vi "KM_file - read-write - list of lines.vi"(7 "read/write control":T1, 9 "header":string, 10 "list of lines IN":string[](array[string]), 11 "file path":path=path "\\\\rus-one\\newdata/data/Ultrasound/Experiment/ProbeTest/Probe10/Hg1201-6-C185-550Cair-3c-83K/sweep3/9w/3366_a.dat") -> (1 "header OUT":string, 2 "list of lines OUT":string[](array[string]))   [LabVIEW 2015]
uses:
  file -- read-write control.ctl
  <vilib>/Utility/file.llb/Read From Spreadsheet File (string).vi
  <vilib>/Utility/file.llb/Write To Spreadsheet File (string).vi
  <vilib>/Utility/file.llb/Write Delimited Spreadsheet (string).vi
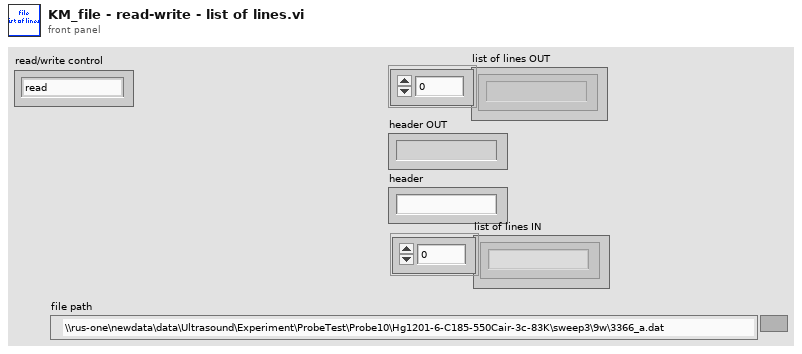
[diagram p1: front panel]
types:
  T1 = typedef "file -- read-write control.ctl" = enum16{"read", "write all", "append one line"}
  T2 = enum16{"open", "replace", "create", "open or create", "replace or create", "replace or create with confirmation"}
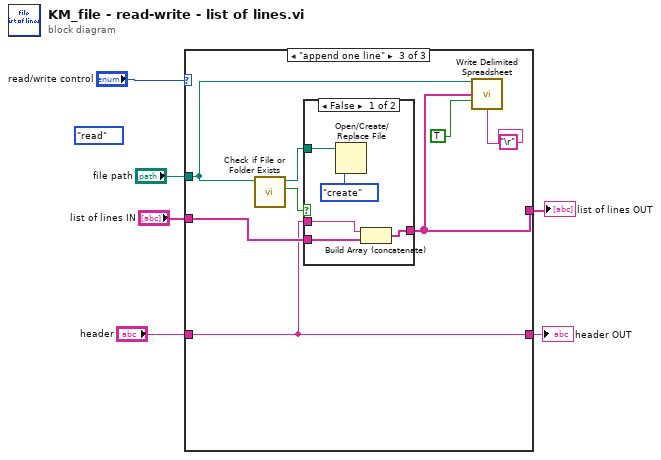
[diagram p0: block diagram]
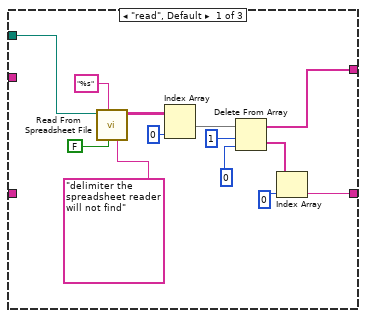
[diagram p2: hidden frame]
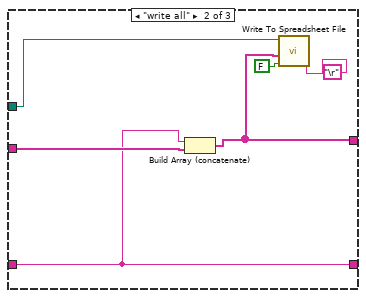
[diagram p3: hidden frame]
diagram:
  (unwired) file_--_read-write_control."read" ("read/write control")
  n1 = case shown="\"append one line\"" "read/write control" {
    tunnel: "file path" -> [w12 w23 w30]
    tunnel: [w8 w21 w26] -> w5
    tunnel: [w7 w20 w28] -> w4
    tunnel: "header" -> [_ w20 w28]
    tunnel: "list of lines IN" -> [_ w22 w29]
    frame "read", Default {
      n2 = call-poly <vilib>:"Read From Spreadsheet File.vi"("delimiter (\\t)"="delimiter the spreadsheet reader will not find" ("delimiter (\\t)"), "transpose (no:F)"=FALSE ("append to file? (new file:F)"), "format (%s)"="%s", "file path (dialog if empty)"=w12) -> ("all rows"=w17:string[][])  [unwired: 3 in, 4 out]
      n3 = Index Array(array=w17, index (col)=0 ("disabled index (col)")) -> (element=w15:string[])  [unwired: 1 in]
      n4 = Delete From Array(array=w15, length=1, index=0) -> (deleted portion=w10:string[], array with subset deleted=w8:string[])
      n5 = Index Array(array=w10, index=0 ("disabled index (col)")) -> (element=w7:string)
    }
    frame "write all" {
      n6 = Build Array (concatenate)(w20, w22) -> (w21:string[])
      n7 = call-poly <vilib>:"Write To Spreadsheet File.vi"("delimiter (\\t)"="\r", "append to file? (new file:F)"=FALSE, "1D data"=w21, "file path (dialog if empty)"=w23) -> ()  [unwired: 4 in, 1 out]
    }
    frame "append one line" {
      n8 = call <vilib>:"Check if File or Folder Exists.vi"("path"=w30) -> ("file or folder exists?"=w31:bool, "dup path"=w27:path)  [unwired: 8 in, 1 out]
      n9 = case shown="False" w31 {
        tunnel: w29 -> [w38 w39]
        tunnel: w28 -> [w37 _]
        tunnel: [w36 w39] -> w26
        tunnel: w27 -> [w35 _]
        frame False {
          n10 = Open/Create/Replace File(file path (use dialog)=w35, operation (0:open)=T2."create") -> ()  [unwired: 4 in, 3 out]
          n11 = Build Array (concatenate)(w37, w38) -> (w36:string[])
        }
        frame True {
        }
      }
      n12 = call-poly <vilib>:"Write Delimited Spreadsheet.vi"("file path (dialog if empty)"=w30, "1D data"=w26, "append to file? (F)"=TRUE ("append to file? (new file:F)"), "delimiter (\\t)"="\r") -> ()  [unwired: 10 in, 2 out]
    }
  }
  "list of lines OUT" <- w5
  "header OUT" <- w4
